vi "9221 8Ch Analog Input.vi"(1 "9221 I/O":T1={"9221 AI0"="NI 9221/AI0", "9221 AI1"="NI 9221/AI1", "9221 AI2"="NI 9221/AI2", "9221 AI3"="NI 9221/AI3", "9221 AI4"="NI 9221/AI4", "9221 AI5"="NI 9221/AI5", "9221 AI6"="NI 9221/AI6", "9221 AI7"="NI 9221/AI7"}) -> (0 "Packets":u64[](array[numeric]))   [LabVIEW 2010]
uses:
  <vilib>/eio/EIONode/EIONode.xnode
  <vilib>/rvi/eio/nirviEIOImplementation/nirviEIOImplementation.xnode
  <vilib>/rvi/eio/common/nirviEmuClasses.ctl
  <vilib>/rvi/eio/common/nirviEmuTemplateMethod_noerrors.vi
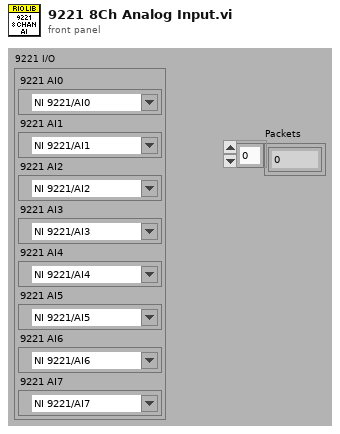
[diagram p1: front panel]
types:
  T1 = cluster{"9221 AI0":refnum<k21>, "9221 AI1":refnum<k21>, "9221 AI2":refnum<k21>, "9221 AI3":refnum<k21>, "9221 AI4":refnum<k21>, "9221 AI5":refnum<k21>, "9221 AI6":refnum<k21>, "9221 AI7":refnum<k21>}
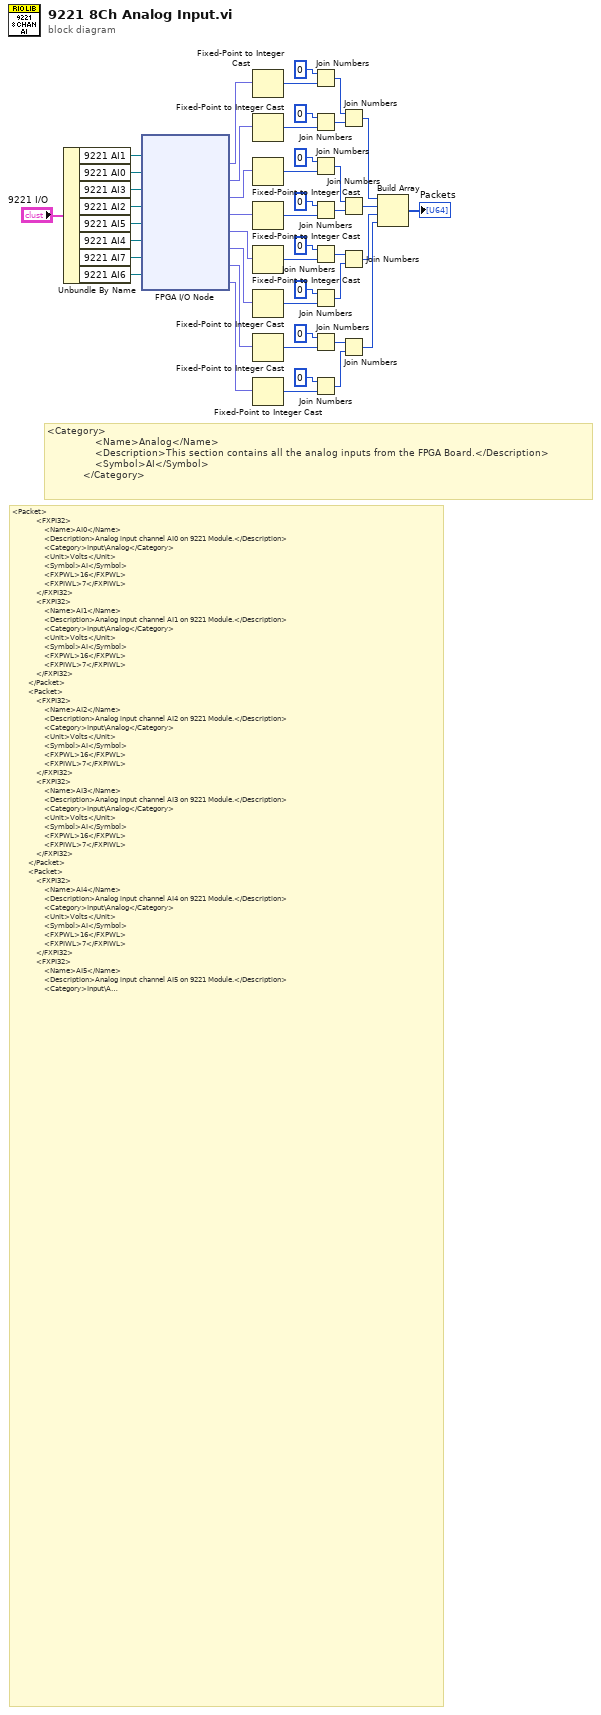
[diagram p0: block diagram]
diagram:
  # "<Category>\n                <Name>Analog</Name>\n                <Description>This section contains all the analog inputs from the FPGA Board.</Description>\n                <Symbol>AI</Symbol>\n            </Category>"
  # "<Packet>\n            <FXPI32>\n                <Name>AI0</Name>\n                <Description>Analog input channel AI0 on 9221 Module.</Description>\n                <Category>Input\\Analog</Category>\n                <Unit>Volts</Unit>\n                <Symbol>AI</Symbol>\n                <FXPWL>16</FXPWL>\n                <FXPIWL>7</FXPIWL>\n            </FXPI32>\n            <FXPI32>\n                <Name>AI1</Name>\n                <Description>Analog input channel AI1 on 9221 Module.</Description>\n                <Category>Input\\Analog</Category>\n                <Unit>Volts</Unit>\n                <Symbol>AI</Symbol>\n                <FXPWL>16</FXPWL>\n                <FXPIWL>7</FXPIWL>\n            </FXPI32>\n        </Packet>\n        <Packet>\n            <FXPI32>\n                <Name>AI2</Name>\n                <Description>Analog input channel AI2 on 9221 Module.</Description>\n                <Category>Input\\Analog</Category>\n                <Unit>Volts</Unit>\n                <Symbol>AI</Symbol>\n                <FXPWL>16</FXPWL>\n                <FXPIWL>7</FXPIWL>\n            </FXPI32>\n            <FXPI32>\n                <Name>AI3</Name>\n                <Description>Analog input channel AI3 on 9221 Module.</Description>\n                <Category>Input\\Analog</Category>\n                <Unit>Volts</Unit>\n                <Symbol>AI</Symbol>\n                <FXPWL>16</FXPWL>\n                <FXPIWL>7</FXPIWL>\n            </FXPI32>\n        </Packet>\n        <Packet>\n            <FXPI32>\n                <Name>AI4</Name>\n                <Description>Analog input channel AI4 on 9221 Module.</Description>\n                <Category>Input\\Analog</Category>\n                <Unit>Volts</Unit>\n                <Symbol>AI</Symbol>\n                <FXPWL>16</FXPWL>\n                <FXPIWL>7</FXPIWL>\n            </FXPI32>\n            <FXPI32>\n                <Name>AI5</Name>\n                <Description>Analog input channel AI5 on 9221 Module.</Description>\n                <Category>Input\\Analog</Category>\n                <Unit>Volts</Unit>\n                <Symbol>AI</Symbol>\n                <FXPWL>16</FXPWL>\n                <FXPIWL>7</FXPIWL>\n            </FXPI32>\n        </Packet>\n        <Packet>\n            <FXPI32>\n                <Name>AI6</Name>\n                <Description>Analog input channel AI6 on 9221 Module.</Description>\n                <Category>Input\\Analog</Category>\n                <Unit>Volts</Unit>\n                <Symbol>AI</Symbol>\n                <FXPWL>16</FXPWL>\n                <FXPIWL>7</FXPIWL>\n            </FXPI32>\n            <FXPI32>\n                <Name>AI7</Name>\n                <Description>Analog input channel AI7 on 9221 Module.</Description>\n                <Category>Input\\Analog</Category>\n                <Unit>Volts</Unit>\n                <Symbol>AI</Symbol>\n                <FXPWL>16</FXPWL>\n                <FXPIWL>7</FXPIWL>\n            </FXPI32>\n        </Packet>"
  n1 = Unbundle By Name("9221 I/O") -> ("9221 AI1"=w42:refnum<k21>, "9221 AI0"=w44:refnum<k21>, "9221 AI3"=w43:refnum<k21>, "9221 AI2"=w45:refnum<k21>, "9221 AI5"=w38:refnum<k21>, "9221 AI4"=w39:refnum<k21>, "9221 AI7"=w40:refnum<k21>, "9221 AI6"=w41:refnum<k21>)
  n2 = xnode "FPGA I/O Node"("FPGA I/O In"=w42, "FPGA I/O In"=w44, "FPGA I/O In"=w43, "FPGA I/O In"=w45, "FPGA I/O In"=w38, "FPGA I/O In"=w39, "FPGA I/O In"=w40, "FPGA I/O In"=w41) -> ("I/O Item"=w8:fxp<+/-,16,7>, "I/O Item"=w7:fxp<+/-,16,7>, "I/O Item"=w6:fxp<+/-,16,7>, "I/O Item"=w5:fxp<+/-,16,7>, "I/O Item"=w4:fxp<+/-,16,7>, "I/O Item"=w3:fxp<+/-,16,7>, "I/O Item"=w2:fxp<+/-,16,7>, "I/O Item"=w1:fxp<+/-,16,7>)  [unwired: 8 out]
  n3 = Fixed-Point to Integer Cast(1:w8) -> (0:w36:i16)
  n4 = Fixed-Point to Integer Cast(1:w7) -> (0:w33:i16)
  n5 = Fixed-Point to Integer Cast(1:w6) -> (0:w30:i16)
  n6 = Fixed-Point to Integer Cast(1:w5) -> (0:w27:i16)
  n7 = Fixed-Point to Integer Cast(1:w4) -> (0:w23:i16)
  n8 = Fixed-Point to Integer Cast(1:w3) -> (0:w20:i16)
  n9 = Fixed-Point to Integer Cast(1:w2) -> (0:w11:i16)
  n10 = Fixed-Point to Integer Cast(1:w1) -> (0:w14:i16)
  n11 = Join Numbers(hi=i16 0, lo=w36) -> ((hi.lo)=w32:u32)
  n12 = Join Numbers(hi=i16 0, lo=w33) -> ((hi.lo)=w31:u32)
  n13 = Join Numbers(hi=i16 0, lo=w30) -> ((hi.lo)=w26:u32)
  n14 = Join Numbers(hi=i16 0, lo=w27) -> ((hi.lo)=w25:u32)
  n15 = Join Numbers(hi=i16 0, lo=w23) -> ((hi.lo)=w19:u32)
  n16 = Join Numbers(hi=i16 0, lo=w20) -> ((hi.lo)=w18:u32)
  n17 = Join Numbers(hi=i16 0, lo=w11) -> ((hi.lo)=w15:u32)
  n18 = Join Numbers(hi=i16 0, lo=w14) -> ((hi.lo)=w16:u32)
  n19 = Join Numbers(hi=w32, lo=w31) -> ((hi.lo)=w37:u64)
  n20 = Join Numbers(hi=w26, lo=w25) -> ((hi.lo)=w24:u64)
  n21 = Join Numbers(hi=w19, lo=w18) -> ((hi.lo)=w17:u64)
  n22 = Join Numbers(hi=w15, lo=w16) -> ((hi.lo)=w10:u64)
  n23 = Build Array(w37, w24, w17, w10) -> (→"Packets":u64[])
